vi "Get column name.vi"(8 "error in (no error)":errorcluster, 11 "Column in":refnum<class "Column Parent.lvclass">) -> (0 "error out":errorcluster, 2 "Column Name":string, 3 "Column out":refnum<class "Column Parent.lvclass">)   [LabVIEW 2020, in "Basic Columns.lvlib" / "Column Parent.lvclass"]
uses:
  Column Parent.lvclass
  Column Configuration/Basic Column Configuration Class/Column Configuration.lvclass
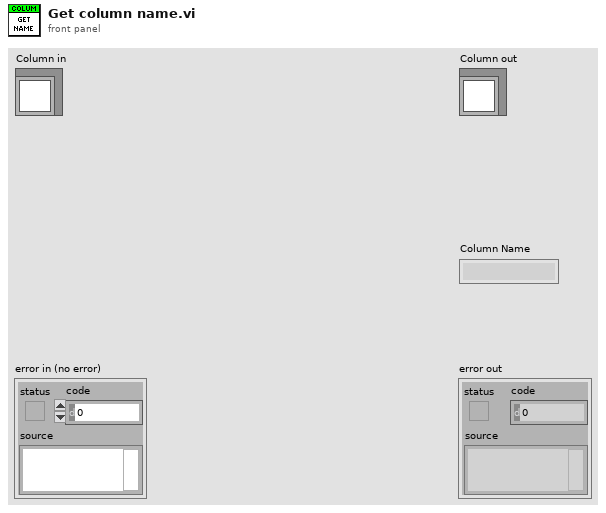
[diagram p1: front panel]
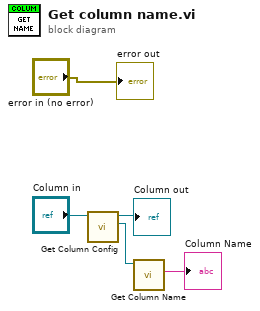
[diagram p0: block diagram]
diagram:
  n1 = call-dynamic "Get Column Config.vi"("Column Parent in"="Column in") -> ("Column Configuration"=w2:refnum<class "Column Configuration.lvclass">, "Column Parent out"=→"Column out":refnum<class "Column Parent.lvclass">)  [unwired: 8 in, 1 out]
  n2 = call-dynamic "Get Column Name.vi"("Basic Column Configuration in"=w2) -> ("Column Name"=→"Column Name":string)  [unwired: 8 in, 2 out]
  "error out" <- "error in (no error)"
